vi "NextState.vi"(8 "error in (no error)":errorcluster, 11 "Queue in":refnum<queue>) -> (0 "error out":errorcluster, 2 "Next State":T1, 3 "Queue out":refnum<queue>)   [LabVIEW 2017, in "Shared Variables CD 2.0 Configuration.lvlib"]
uses:
  Shared Variables CD 2.0 Configuration.lvlib
  Channel Configuration States.ctl
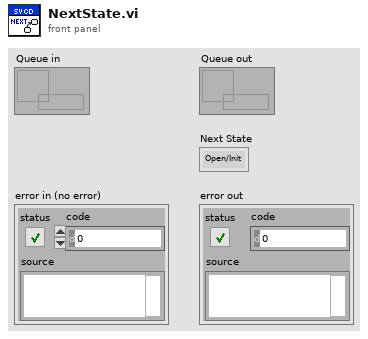
[diagram p1: front panel]
types:
  T1 = typedef "Shared Variables CD 2.0 Configuration.lvlib/Channel Configuration States.ctl" = enum16{"Open/Init", "Start Update", "Get VS Channels", "Get Available Ch from Target", "Wait On User Action", "Update Target Tree", "Update VS Trees", "Update Done", "Create VS Channels", "Remove VS Channels", "Error", "Close"}
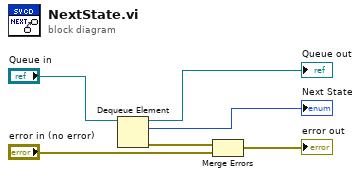
[diagram p0: block diagram]
diagram:
  n1 = Dequeue Element(queue="Queue in") -> (queue out=→"Queue out":refnum<queue>, element=→"Next State":T1, error out=w2:errorcluster)  [unwired: 2 in, 1 out]
  n2 = Merge Errors(w2, "error in (no error)") -> (→"error out":errorcluster)
